vi "PruebaAutoR-Seq.vi"() -> ()   [LabVIEW 2014, in "MSX-E3701.lvlib"]
uses:
  MSX-E3701.lvlib
  DriverMasterSync/build/DriverMasterSync.lvlibp/Modules/HAL/TypeDefs/HAL Config Data.ctl
  DriverMasterSync/build/DriverMasterSync.lvlibp/APIs/Data Queue/Acquisition Data 1 Sample Cluster.ctl
  DriverMasterSync/build/DriverMasterSync.lvlibp/APIs/Data Queue/Control Data Cluster.ctl
  MSX-E3701Class/MSX-E3701.lvclass
  DriverMasterSync/build/DriverMasterSync.lvlibp
  DriverMasterSync/build/DriverMasterSync.lvlibp/APIs/Data Queue/WINFAS 2 Data Queue.lvlib
panel:
  out "error out 2":errorcluster
  out "Array 2":T1[](array[typedef])
  out "Array":T2[](array[typedef])
  out "TDX":sgl[][](array[numeric]) format="%#.5f"
  out "Muestras por seg":dbl
  out "Segundos":dbl
  out "Muestras":i32
  out "error out":errorcluster
  in  "stop 2":bool
  out "HAL Config Data":T3
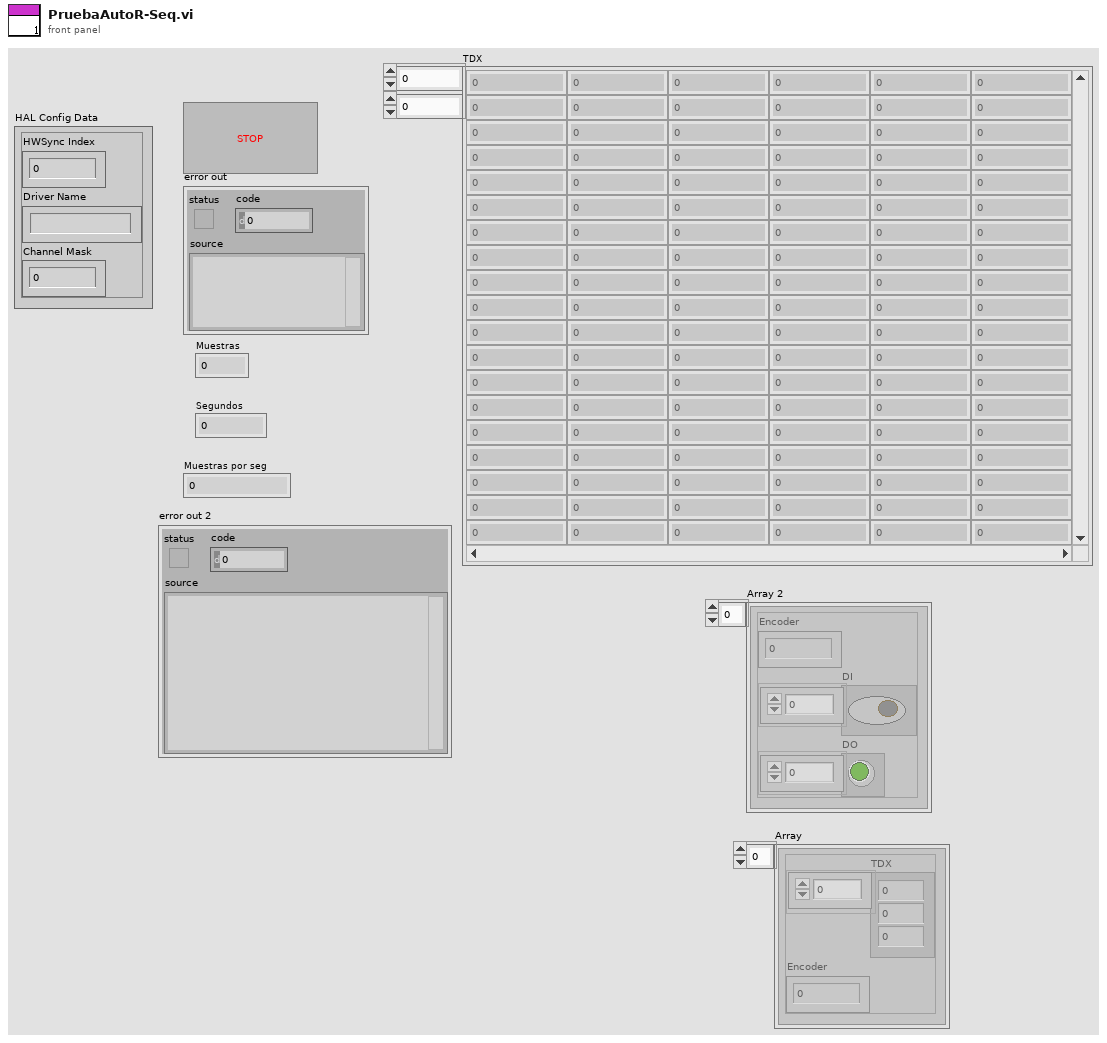
[diagram p1: front panel]
types:
  T1 = typedef "DriverMasterSync.lvlibp/WINFAS 2 Data Queue.lvlib/Control Data Cluster.ctl" = cluster{"Encoder":sgl, "DI":bool[], "DO":bool[]}
  T2 = typedef "DriverMasterSync.lvlibp/WINFAS 2 Data Queue.lvlib/Acquisition Data 1 Sample Cluster.ctl" = cluster{"TDX":sgl[], "Encoder":sgl}
  T3 = typedef "DriverMasterSync.lvlibp/HAL Config Data.ctl" = cluster{"HWSync Index":u32, "Driver Name":string, "Channel Mask":u64}
  T4 = typedef "DriverMasterSync.lvlibp/WINFAS 2 Data Queue.lvlib/Acquisition Data Cluster.ctl" = T2[]
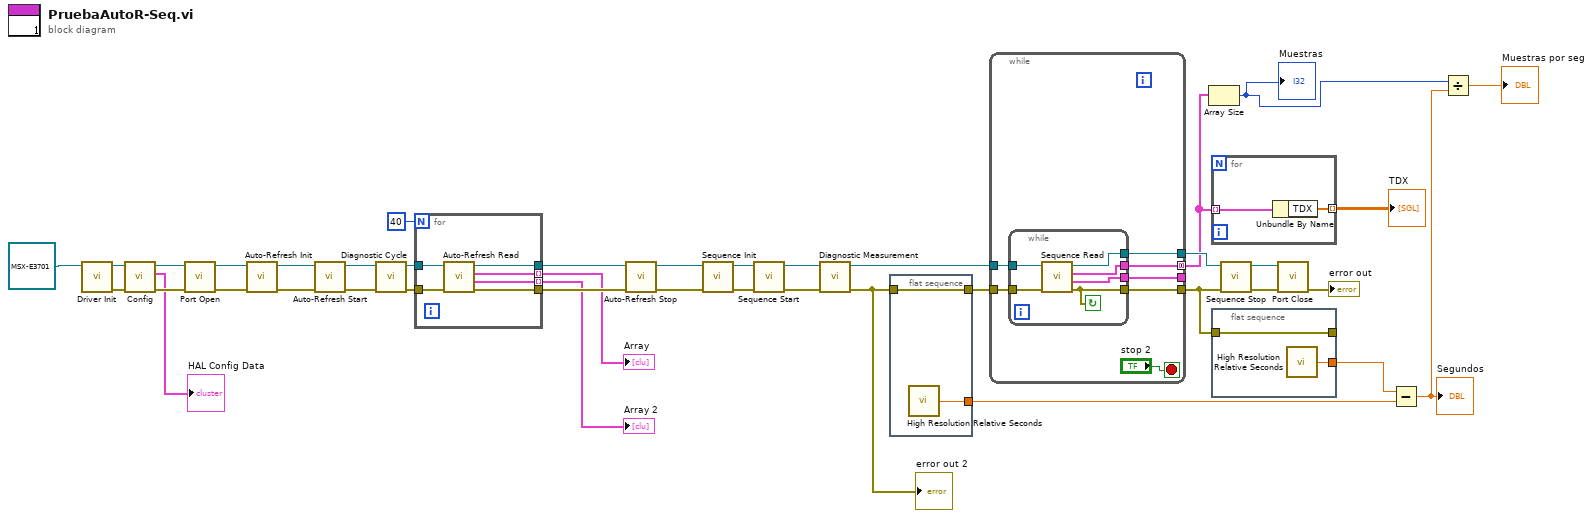
[diagram p0: block diagram]
diagram:
  n1 = call-dynamic "Driver Init.vi"("MSX-E3701 in"=refnum<class "MSX-E3701.lvclass"> refnum) -> ("error out"=w33:errorcluster, "MSX-E3701 out"=w34:refnum<class "MSX-E3701.lvclass">)  [unwired: 9 in]
  n2 = call-dynamic "Config.vi"("error in (no error)"=w33, "MSX-E3701 in"=w34) -> ("error out"=w37:errorcluster, "HAL Config Data"=→"HAL Config Data":T3, "MSX-E3701 out"=w40:refnum<class "MSX-E3701.lvclass">)  [unwired: 7 in]
  n3 = call-dynamic "Port Open.vi"("error in (no error)"=w37, "MSX-E3701 in"=w40) -> ("error out"=w36:errorcluster, "MSX-E3701 out"=w39:refnum<class "MSX-E3701.lvclass">)  [unwired: 8 in]
  n4 = call-dynamic "Auto-Refresh Init.vi"("error in (no error)"=w36, "MSX-E3701 in"=w39) -> ("error out"=w35:errorcluster, "MSX-E3701 out"=w38:refnum<class "MSX-E3701.lvclass">)  [unwired: 8 in]
  n5 = call-dynamic "Auto-Refresh Start.vi"("error in (no error)"=w35, "MSX-E3701 in"=w38) -> ("error out"=w29:errorcluster, "MSX-E3701 out"=w30:refnum<class "MSX-E3701.lvclass">)  [unwired: 8 in]
  n6 = call-dynamic "Diagnostic Cycle.vi"("error in (no error)"=w29, "MSX-E3701 in"=w30) -> ("error out"=w12:errorcluster, "MSX-E3701 out"=w13:refnum<class "MSX-E3701.lvclass">)  [unwired: 8 in]
  n7 = for {
    N: 40 -> [_]
    tunnel: [w42] -> w8 mode=indexing
    tunnel: [w41] -> w7 mode=indexing
    tunnel: w13 -> [w46]
    tunnel: [w44] -> w11
    tunnel: w12 -> [w45]
    tunnel: [w43] -> w10
    n8 = call-dynamic "Auto-Refresh Read.vi"("error in (no error)"=w45, "MSX-E3701 in"=w46) -> ("error out"=w43:errorcluster, "Control Data"=w41:T1, "1 Sample"=w42:T2, "MSX-E3701 out"=w44:refnum<class "MSX-E3701.lvclass">)  [unwired: 6 in]
  }
  "Array" <- w8
  "Array 2" <- w7
  n9 = call-dynamic "Auto-Refresh Stop.vi"("error in (no error)"=w10, "MSX-E3701 in"=w11) -> ("error out"=w5:errorcluster, "MSX-E3701 out"=w6:refnum<class "MSX-E3701.lvclass">)  [unwired: 8 in]
  n10 = call-dynamic "Sequence Init.vi"("error in (no error)"=w5, "MSX-E3701 in"=w6) -> ("error out"=w28:errorcluster, "MSX-E3701 out"=w24:refnum<class "MSX-E3701.lvclass">)  [unwired: 8 in]
  n11 = call-dynamic "Sequence Start.vi"("error in (no error)"=w28, "MSX-E3701 in"=w24) -> ("error out"=w2:errorcluster, "MSX-E3701 out"=w3:refnum<class "MSX-E3701.lvclass">)  [unwired: 8 in]
  n12 = call-dynamic "Diagnostic Measurement.vi"("error in (no error)"=w2, "MSX-E3701 in"=w3) -> ("error out"=w1:errorcluster, "MSX-E3701 out"=w4:refnum<class "MSX-E3701.lvclass">)  [unwired: 8 in]
  "error out 2" <- w1
  n13 = flat-sequence {
    tunnel: [w48] -> w22
    tunnel: w1 -> [w48]
    tunnel: [w47] -> w19
    frame #0 {
      n14 = call <vilib>:"High Resolution Relative Seconds.vi"() -> ("relative seconds"=w47:dbl)
    }
  }
  n15 = while {
    tunnel: w22 -> [w55]
    tunnel: [w54] -> w21
    tunnel: w4 -> [w52]
    tunnel: [w53] -> w25
    tunnel: [w50] -> w15 mode=concatenating
    tunnel: [w49] -> _
    stop <- "stop 2" stop-if-true
    n16 = while {
      tunnel: w55 -> [w61]
      tunnel: [w58] -> w54
      tunnel: w52 -> [w59]
      tunnel: [w60] -> w53
      tunnel: [w57] -> w50
      tunnel: [w56] -> w49
      stop <- w58 continue-if-true
      n17 = call-dynamic "Sequence Read.vi"("error in (no error)"=w61, "MSX-E3701 in"=w59) -> ("error out"=w58:errorcluster, "Control Data"=w56:T1, "Acquisition Data"=w57:T4, "MSX-E3701 out"=w60:refnum<class "MSX-E3701.lvclass">)  [unwired: 6 in]
    }
  }
  n18 = Array Size(array=w15) -> (size(s)=w14:i32)
  "Muestras" <- w14
  n19 = for {
    tunnel: w15 -> [w63] mode=indexing
    tunnel: [w62] -> w16 mode=indexing
    n20 = Unbundle By Name(w63) -> ("TDX"=w62:sgl[])
  }
  "TDX" <- w16
  n21 = flat-sequence {
    tunnel: [w65] -> _
    tunnel: w21 -> [w65]
    tunnel: [w64] -> w20
    frame #0 {
      n22 = call <vilib>:"High Resolution Relative Seconds.vi"() -> ("relative seconds"=w64:dbl)
    }
  }
  n23 = call-dynamic "Sequence Stop.vi"("error in (no error)"=w21, "MSX-E3701 in"=w25) -> ("error out"=w27:errorcluster, "MSX-E3701 out"=w26:refnum<class "MSX-E3701.lvclass">)  [unwired: 8 in]
  n24 = call-dynamic "Port Close.vi"("error in (no error)"=w27, "MSX-E3701 in"=w26) -> ("error out"=→"error out":errorcluster)  [unwired: 8 in, 1 out]
  n25 = Subtract(x=w20, y=w19) -> (x-y=w18:dbl)
  "Segundos" <- w18
  n26 = Divide(x=w14, y=w18) -> (x/y=→"Muestras por seg":dbl)
